vi "_interfacebrowser build tree table in CSM-VI mode.vi"(6 "Config Path":path, 8 "Error in":errorcluster caption="Error in (no error)", 9 "Opton:All-CSM-VIs":bool) -> (0 "Error out":errorcluster, 2 "Type":string[](array[string]), 3 "Tree Table":string[][](array[string]))   [LabVIEW 2017, in "interfacebrowser.lvlib"]
uses:
  interfacebrowser.lvlib
  _csmHelper/API with lvcsm Support/CSM-Helper API with lvcsm Support.lvlib
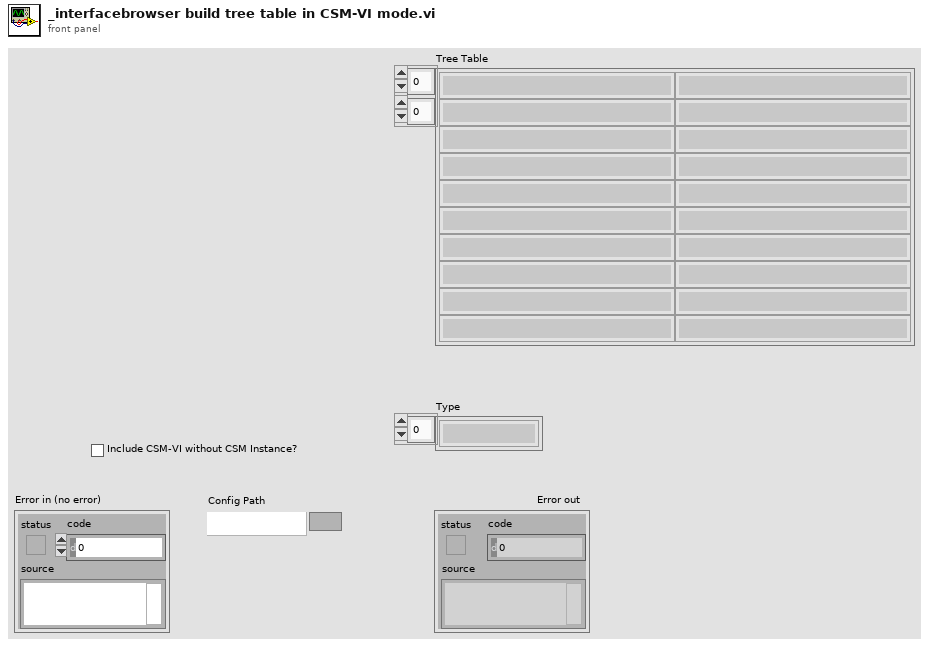
[diagram p1: front panel]
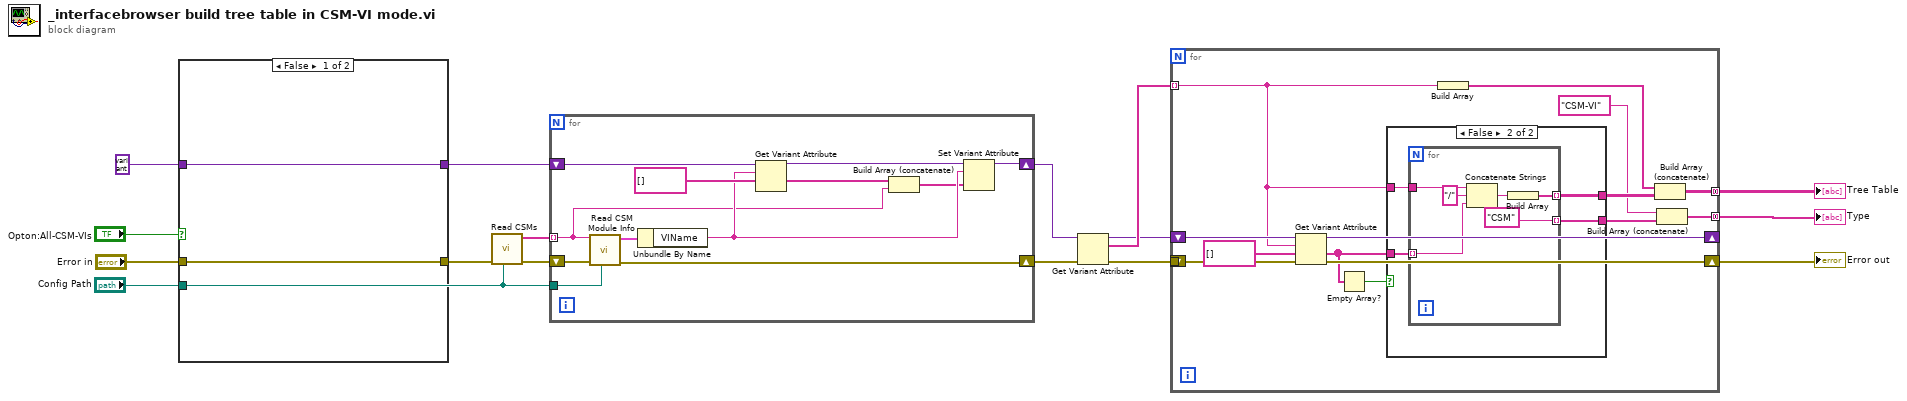
[diagram p0: block diagram]
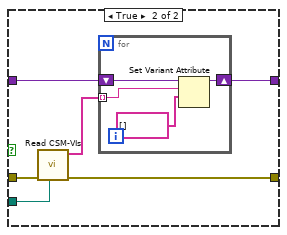
[diagram p2: hidden frame]
diagram:
  n1 = case shown="False" "Opton:All-CSM-VIs" {
    tunnel: "Error in" -> [w18 w24]
    tunnel: [w18 w23] -> w5
    tunnel: variant -> [w17 w22]
    tunnel: [w17 w21] -> w3
    tunnel: "Config Path" -> [_ w19]
    frame False {
    }
    frame True {
      n2 = call "Read CSM-VIs.vi"("Config Path"=w19, "Error in"=w24) -> ("Error out"=w23:errorcluster, "Array"=w20:string[])  [unwired: 8 in]
      n3 = for {
        shift-right: [w27] -> w21
        shift-left: w22 -> [w28]
        tunnel: w20 -> [w25] mode=indexing
        n4 = Set Variant Attribute(Variant=w28, name=w25, value=string[] [] ("Delimiter")) -> (Variant out=w27:variant)  [unwired: 1 in, 2 out]
      }
    }
  }
  n5 = call "Read CSMs.vi"("Config Path"="Config Path", "Error in"=w5) -> ("Error out"=w14:errorcluster, "Array"=w16:string[])  [unwired: 8 in]
  n6 = for {
    tunnel: w16 -> [w29] mode=indexing
    tunnel: "Config Path" -> [w38]
    shift-right: [w37] -> w13
    shift-left: w14 -> [w39]
    shift-right: [w33] -> w12
    shift-left: w3 -> [w36]
    n7 = call "Read CSM Module Info.vi"("Config Path"=w38, "error in (no error)"=w39, "CSM Name"=w29) -> ("error out"=w37:errorcluster, "Cluster"=w40:cluster{"VIName":string})  [unwired: 7 in]
    n8 = Unbundle By Name(w40) -> ("VIName"=w32:string)
    n9 = Get Variant Attribute(Variant=w36, name=w32, default value (empty Variant)=string[] [] ("Delimiter")) -> (duplicate Variant=w34:variant, value=w31:string[])  [unwired: 1 in, 2 out]
    n10 = Build Array (concatenate)(w31, w29) -> (w30:string[])
    n11 = Set Variant Attribute(Variant=w34, name=w32, value=w30) -> (Variant out=w33:variant)  [unwired: 1 in, 2 out]
  }
  n12 = Get Variant Attribute(Variant=w12, error in=w13) -> (duplicate Variant=w10:variant, names=w11:string[], error out=w9:errorcluster)  [unwired: 2 in, 1 out]
  n13 = for {
    tunnel: w11 -> [w48] mode=indexing
    shift-right: [w52] -> _
    shift-left: w10 -> [w53]
    tunnel: w9 -> [w51]
    shift-right: [w50] -> w8
    shift-left: _ -> [_]
    tunnel: [w47] -> w7 mode=concatenating
    tunnel: [w45] -> w6 mode=concatenating
    n14 = Get Variant Attribute(Variant=w53, name=w48, default value (empty Variant)=string[] [] ("Delimiter"), error in=w51) -> (duplicate Variant=w52:variant, value=w42:string[], error out=w50:errorcluster)  [unwired: 1 out]
    n15 = Empty Array?(array=w42) -> (empty?=w41:bool)
    n16 = case shown="False" w41 {
      tunnel: [_ w58] -> w49
      tunnel: w48 -> [_ w57]
      tunnel: [_ w56] -> w44
      tunnel: w42 -> [_ w55]
      frame True {
      }
      frame False {
        n17 = for {
          tunnel: w57 -> [w64]
          tunnel: w55 -> [w63] mode=indexing
          tunnel: [w60] -> w58 mode=indexing
          tunnel: ["CSM" ("string")] -> w56 mode=indexing
          n18 = Concatenate Strings(w64, "/" ("string"), w63) -> (w61:string)
          n19 = Build Array(w61) -> (w60:string[])
        }
      }
    }
    n20 = Build Array(w48) -> (w46:string[])
    n21 = Build Array (concatenate)(w46, w49) -> (w47:string[][])
    n22 = Build Array (concatenate)("CSM-VI" ("string"), w44) -> (w45:string[])
  }
  "Type" <- w6
  "Tree Table" <- w7
  "Error out" <- w8
